vi "TESTJOG.vi"() -> ()   [LabVIEW 2016]
uses:
  <vilib>/vision/driver/NI_Vision_Acquisition_Software.lvlib
panel:
  in  "stop 2":bool
  out "Image Out":T1(plugin-control)
  in  "Camera Name":refnum<k21>="cam0" caption="IMAQdx Session"
  in  "Jog step size":T2={"X [mm]"=0.001, "Y [mm]"=0.001, "Z [mm]"=0.001}
  in  "- move":bool
  in  "+ move":bool
  in  "Axis name":string(combo)
  in  "stop":bool
  out "Moving":bool
  out "Stave origin":T2
  out "Current stage position [mm]":cluster{"X":dbl, "Y":dbl, "Z":dbl}
  in  "Axis Speeds":T3={"X [mm/s]"=10.0, "Y [mm/s]"=10.0, "Z [mm/s]"=10.0}
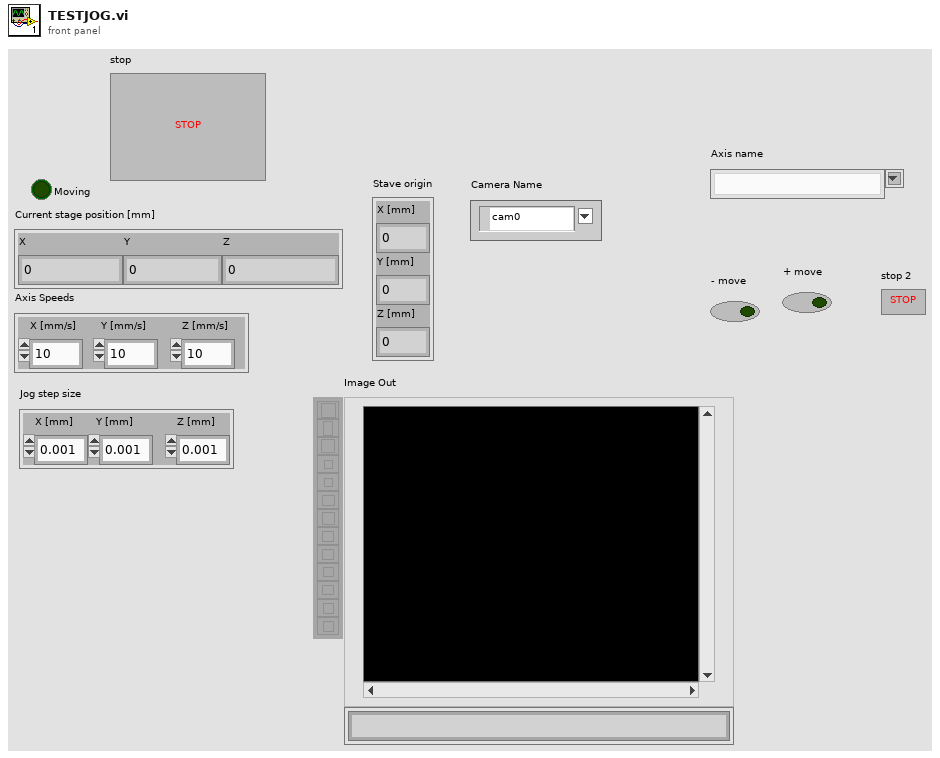
[diagram p1: front panel]
types:
  T1 = typedef "IMAQ Image.ctl" = refnum<image>
  T2 = cluster{"X [mm]":dbl, "Y [mm]":dbl, "Z [mm]":dbl}
  T3 = cluster{"X [mm/s]":dbl, "Y [mm/s]":dbl, "Z [mm/s]":dbl}
  T4 = cluster{"Final X":dbl, "Final Y":dbl, "Final Z":dbl}
  T5 = typedef "IMAQdx.ctl" = refnum<k21>
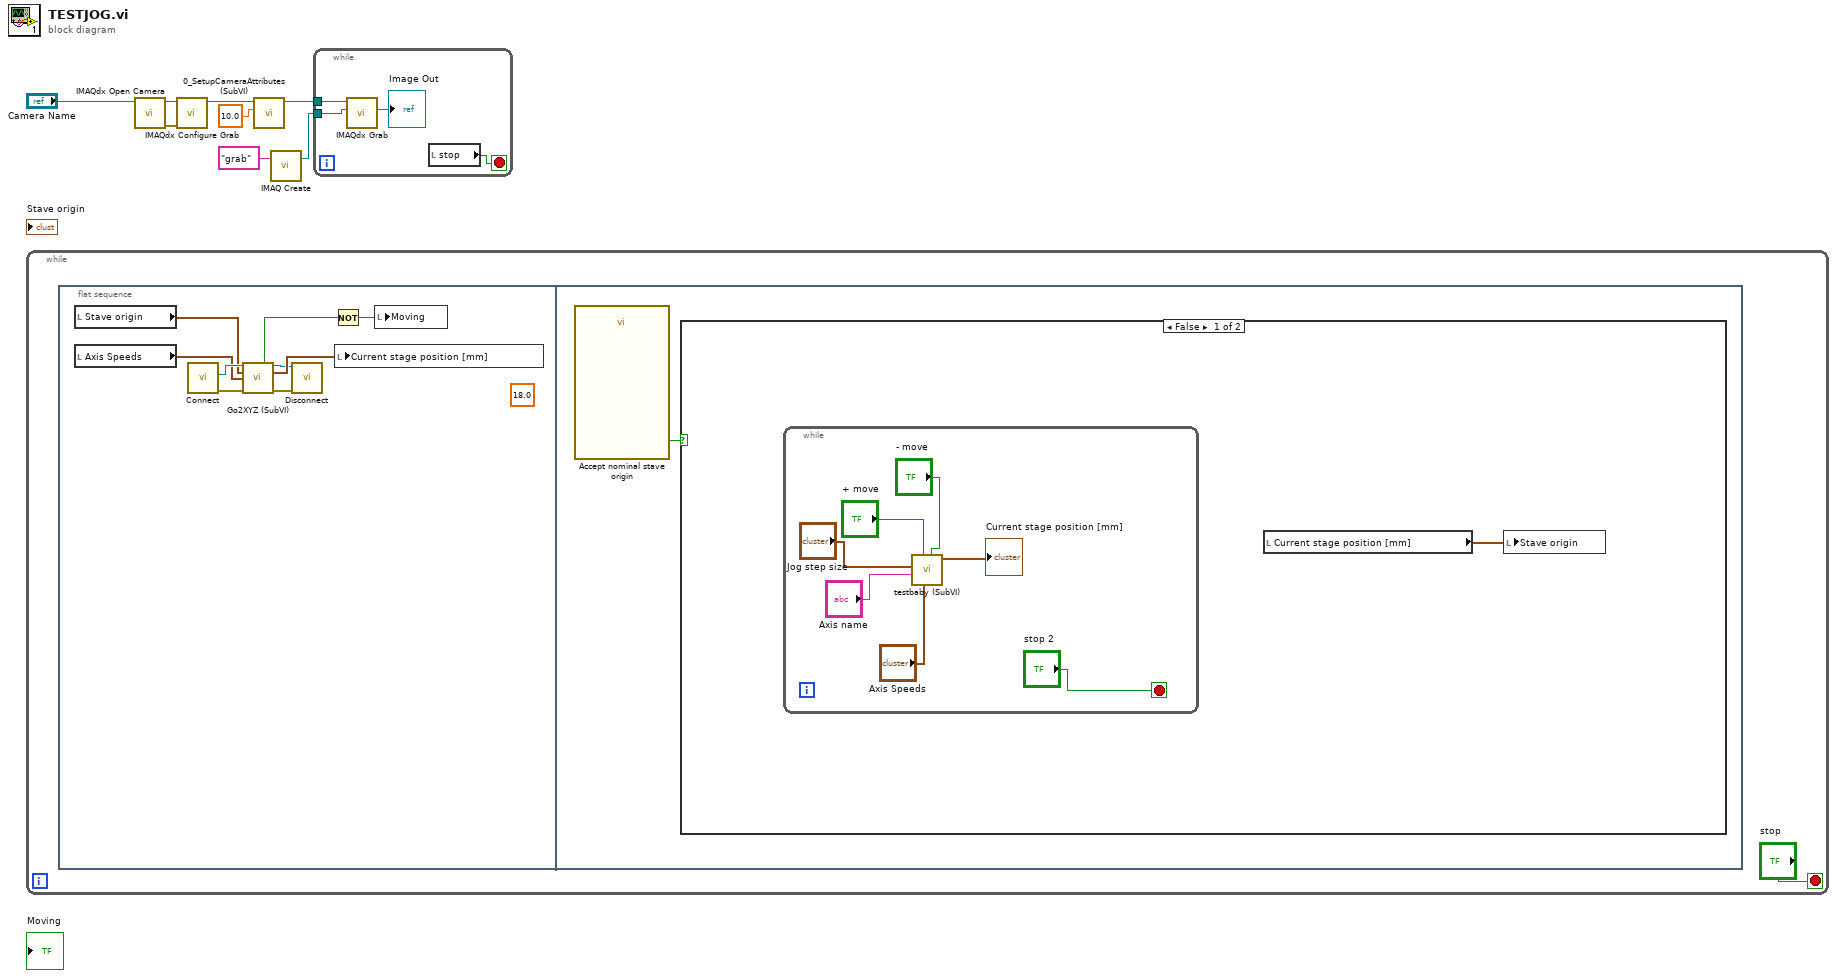
[diagram p0: block diagram]
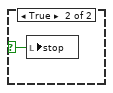
[diagram p2: hidden frame]
diagram:
  n1 = while {
    stop <- "stop" stop-if-true
    n2 = flat-sequence {
      frame #0 {
        (unwired) 18.0 ("Camera gain")
        n3 = local read "Stave origin"() -> (w11:T2)
        n4 = local read "Axis Speeds"() -> (w10:T3)
        n5 = call "Connect.vi"() -> ("error out"=w15:errorcluster, "controller"=w16:refnum<k24>)  [unwired: 10 in]
        n6 = call "Go2XYZ (SubVI).vi"(".NET Refnum in"=w16, "Go to Coordinates"=w11, "Axis Speeds"=w10, "error in (no error)"=w15) -> ("completed"=w17:bool, ".NET Refnum out"=w12:refnum<k24>, "Final Position"=w13:T4, "error out"=w14:errorcluster)  [unwired: 7 in, 1 out]
        n7 = call "Disconnect.vi"("error in (no error)"=w14, "controller"=w12) -> ()  [unwired: 9 in, 1 out]
        n8 = Not(x=w17) -> (.not. x?=w18:bool)
        n9 = local write "Current stage position [mm]"(w13) -> ()
        n10 = local write "Moving"(w18) -> ()
      }
      frame #1 {
        n11 = call "Accept nominal stave origin"() -> ("Accept stave origin"=w19:bool)  [unwired: 17 in, 2 out]
        n12 = case shown="False" w19 {
          selector: w19 -> [_ w28]
          frame False {
            n13 = while {
              stop <- "stop 2" stop-if-true
              n14 = call "testbaby (SubVI).vi"("- move"="- move", "Axis Speeds"="Axis Speeds", "+ move"="+ move", "Axis name"="Axis name", "Jog step size"="Jog step size") -> ("Current stage position [mm]"=→"Current stage position [mm]":cluster{"X":dbl, "Y":dbl, "Z":dbl})  [unwired: 6 in]
            }
            n15 = local read "Current stage position [mm]"() -> (w20:cluster{"X":dbl, "Y":dbl, "Z":dbl})
            n16 = local write "Stave origin"(w20) -> ()
          }
          frame True {
            n17 = local write "stop"(w28) -> ()
          }
        }
      }
    }
  }
  n18 = call <vilib>:"IMAQdx Open Camera.vi"("Session In"="Camera Name") -> ("error out"=w7:errorcluster, "Session Out"=w8:T5)  [unwired: 2 in, 7 out]
  n19 = call <vilib>:"IMAQdx Configure Grab.vi"("error in"=w7, "Session In"=w8) -> ("Session Out"=w3:T5)  [unwired: 9 out]
  n20 = call "0_SetupCameraAttributes (SubVI).vi"("Gain"=10.0, "Camera session in"=w3) -> ("Camera session out"=w1:T5)  [unwired: 8 in, 1 out]
  n21 = call "IMAQ Create"("Image Name"="grab") -> ("New Image"=w2:T1)  [unwired: 4 in, 1 out]
  n22 = while {
    tunnel: w2 -> [w31]
    tunnel: w1 -> [w30]
    stop <- w32 stop-if-true
    n23 = call <vilib>:"IMAQdx Grab.vi"("Image In"=w31, "Session In"=w30) -> ("Image Out"=→"Image Out":T1)  [unwired: 2 in, 7 out]
    n24 = local read "stop"() -> (w32:bool)
  }
